vi "GetReferenceByUID.vi"(3 "error in (no error)":errorcluster, 4 "objectClass":string="GObject", 5 "UID":i32, 6 "targetVI":refnum<vi>) -> (0 "error out":errorcluster, 1 "refNum":refnum<vi>, 2 "dup targetVI":refnum<vi>)   [LabVIEW 2013]
uses:
  <vilib>/Utility/traverseref.llb/TRef TravTarget.ctl
  <vilib>/Utility/traverseref.llb/VI Scripting - Traverse.lvlib
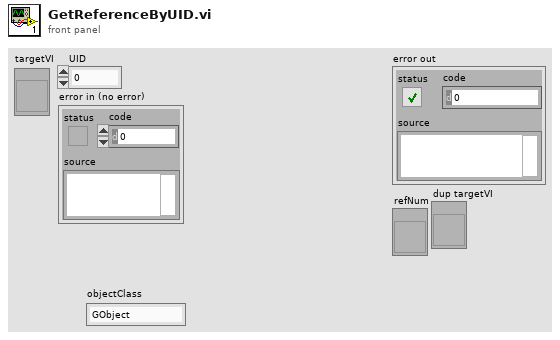
[diagram p1: front panel]
types:
  T1 = typedef "TRef TravTarget.ctl" = enum16{"FP", "BD", "Other"}
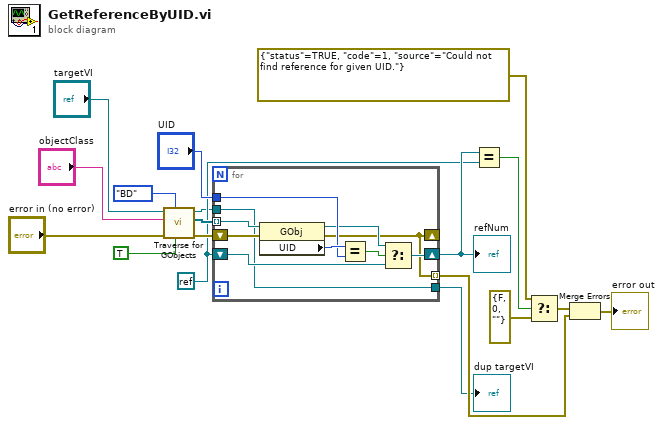
[diagram p0: block diagram]
diagram:
  w11 = refnum<k0> refnum
  n1 = call <vilib>:"Traverse for GObjects.vi"("Traverse Generated Code (F)"=TRUE, "Traverse Target"=TRef_TravTarget."BD", "error in (no error)"="error in (no error)", "Class Name"="objectClass", "VI Refnum"="targetVI") -> ("error out"=w14:errorcluster, "References"=w15:refnum<vi>[], "dup VI Refnum"=w3:refnum<vi>)  [unwired: 3 in, 1 out]
  n2 = for {
    tunnel: w15 -> [w28] mode=indexing
    tunnel: "UID" -> [w25]
    shift-right: [w23] -> w12
    shift-left: w11 -> [w21]
    shift-right: [w20] -> _
    shift-left: w14 -> [w27]
    tunnel: [w20] -> w7 mode=indexing
    tunnel: [w19] -> w2
    tunnel: w3 -> [w19]
    n3 = property class="GObj"(reference=w28, error in=w27) -> (reference out=w22:refnum<vi>, error out=w20:errorcluster, "UID"=w26:i32)
    n4 = Equal?(x=w26, y=w25) -> (x = y?=w24:bool)
    n5 = Select(t=w22, s=w24, f=w21) -> (s? t:f=w23:refnum<vi>)
  }
  "refNum" <- w12
  "dup targetVI" <- w2
  n6 = Equal?(x=w12, y=w11) -> (x = y?=w10:bool)
  n7 = Select(t=errorcluster {"status"=TRUE, "code"=1, "source"="Could not find reference for given UID."}, s=w10, f=errorcluster {"status"=FALSE, "code"=0, "source"=""}) -> (s? t:f=w6:errorcluster)
  n8 = Merge Errors(w6, w7) -> (→"error out":errorcluster)
